vi "Replace Non printable chars.vi"(11 "Value":string) -> (3 "trimmed string":string)   [LabVIEW 2020]
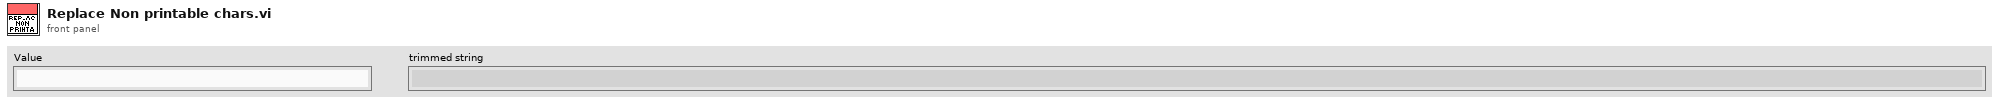
[diagram p1: front panel]
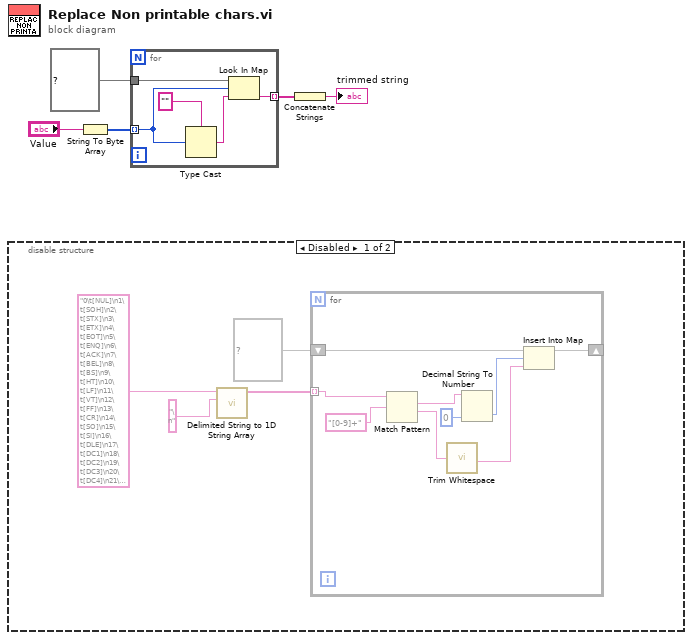
[diagram p0: block diagram]
diagram:
  n1 = disable-structure shown="Disabled" {
    frame Disabled {
      n2 = call <vilib>:"Delimited String to 1D String Array.vi"("delimiter"="\n", "delimited string"="0\t[NUL]\n1\t[SOH]\n2\t[STX]\n3\t[ETX]\n4\t[EOT]\n5\t[ENQ]\n6\t[ACK]\n7\t[BEL]\n8\t[BS]\n9\t[HT]\n10\t[LF]\n11\t[VT]\n12\t[FF]\n13\t[CR]\n14\t[SO]\n15\t[SI]\n16\t[DLE]\n17\t[DC1]\n18\t[DC2]\n19\t[DC3]\n20\t[DC4]\n21\t[NAK]\n22\t[SYN]\n23\t[ETB]\n24\t[CAN]\n25\t[EM]\n26\t[SUB]\n27\t[ESC]\n28\t[FS]\n29\t[GS]\n30\t[RS]\n31\t[US]\n127\t[DEL]") -> ("string array"=w8:string[])  [unwired: 9 in]
      n3 = for {
        tunnel: w8 -> [w18] mode=indexing
        shift-right: [w14] -> _
        shift-left: map{u8, string} {} ("map") -> [w15]
        w11 = u8 0 ("default (0 U32)")
        n4 = Match Pattern(string=w18, regular expression="[0-9]+") -> (match substring=w10:string, after substring=w16:string)  [unwired: 1 in, 2 out]
        n5 = call <vilib>:"Trim Whitespace.vi"("string"=w16) -> ("trimmed string"=w12:string)  [unwired: 1 in]
        n6 = Decimal String To Number(string=w10, offset=w11, default (0L)=w11) -> (number=w13:u8)  [unwired: 1 out]
        n7 = Insert Into Map(map in=w15, key=w13, value=w12) -> (map out=w14:map{u8, string})  [unwired: 2 out]
      }
    }
    frame Enabled {
    }
  }
  n8 = String To Byte Array(string="Value") -> (unsigned byte array=w5:u8[])
  n9 = for {
    tunnel: w5 -> [w21] mode=indexing
    tunnel: map{u8, string} {0="[NUL]", 1="[SOH]", 2="[STX]", 3="[ETX]", 4="[EOT]", 5="[ENQ]", 6="[ACK]", 7="[BEL]", 8="[BS]", 9="[HT]", 10="[LF]", 11="[VT]", 12="[FF]", 13="[CR]", 14="[SO]", 15="[SI]", 16="[DLE]", 17="[DC1]", 18="[DC2]", 19="[DC3]", 20="[DC4]", 21="[NAK]", 22="[SYN]", 23="[ETB]", 24="[CAN]", 25="[EM]", 26="[SUB]", 27="[ESC]", 28="[FS]", 29="[GS]", 30="[RS]", 31="[US]", 127="[DEL]"} ("map") -> [w23]
    tunnel: [w19] -> w4 mode=indexing
    n10 = Type Cast(type="", x=w21) -> (*(type *) &x=w20:string)
    n11 = Look In Map(map=w23, key=w21, default value=w20) -> (value=w19:string)  [unwired: 1 out]
  }
  n12 = Concatenate Strings(w4) -> (→"trimmed string":string)
